vi "Data Format.vi"(9 "Table":refnum<vi>) -> (0 "title":string[](array[string]), 2 "Data":string[](array[string]))   [LabVIEW 2017]
panel:
  out "Error_Description":string
  out "Table":string[][](array[string])
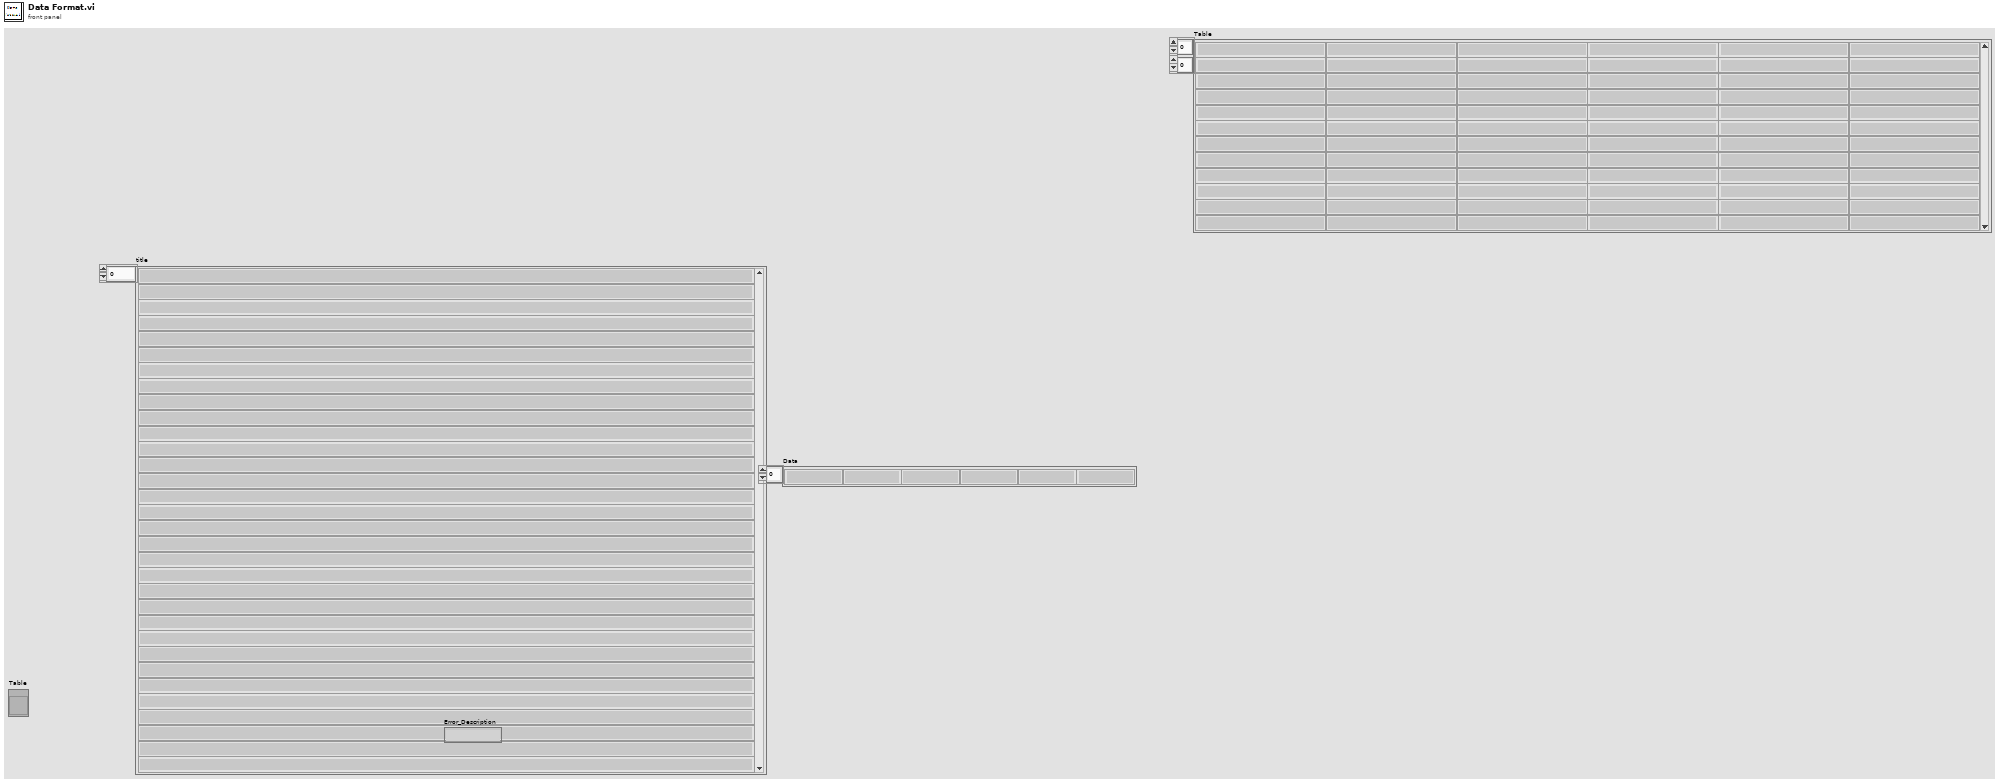
[diagram p1: front panel]
types:
  T1 = typedef "HD Config.ctl" = cluster{" PC":cluster{"PC Address":u8[], "PC Port":i32}, "FCO":cluster{"COM":refnum<visa-resource-name>, "Baudrate":u32}, "DC Power ":cluster{"COM":refnum<visa-resource-name>, "Baudrate":u32}, "PW3336":cluster{"COM":refnum<visa-resource-name>, "Baudrate":u32}, "Lefoo":cluster{"COM":refnum<visa-resource-name>, "Baudrate":u32}, "Tempt&Hum":cluster{"COM":refnum<visa-resource-name>, "Baudrate":u32}, "DIPC":cluster{"COM":refnum<visa-resource-name>}, "Daemon":cluster{"IP Address":string, "Port":u16, "Retry":u16}, "NFC_Cmd":cluster{"COM":refnum<visa-resource-name>, "Baudrate":u32}, "Fail_resume_mode":bool, "GRR":bool, "NFC _Serial":cluster{"COM":refnum<visa-resource-name>, "Baudrate":u32}}
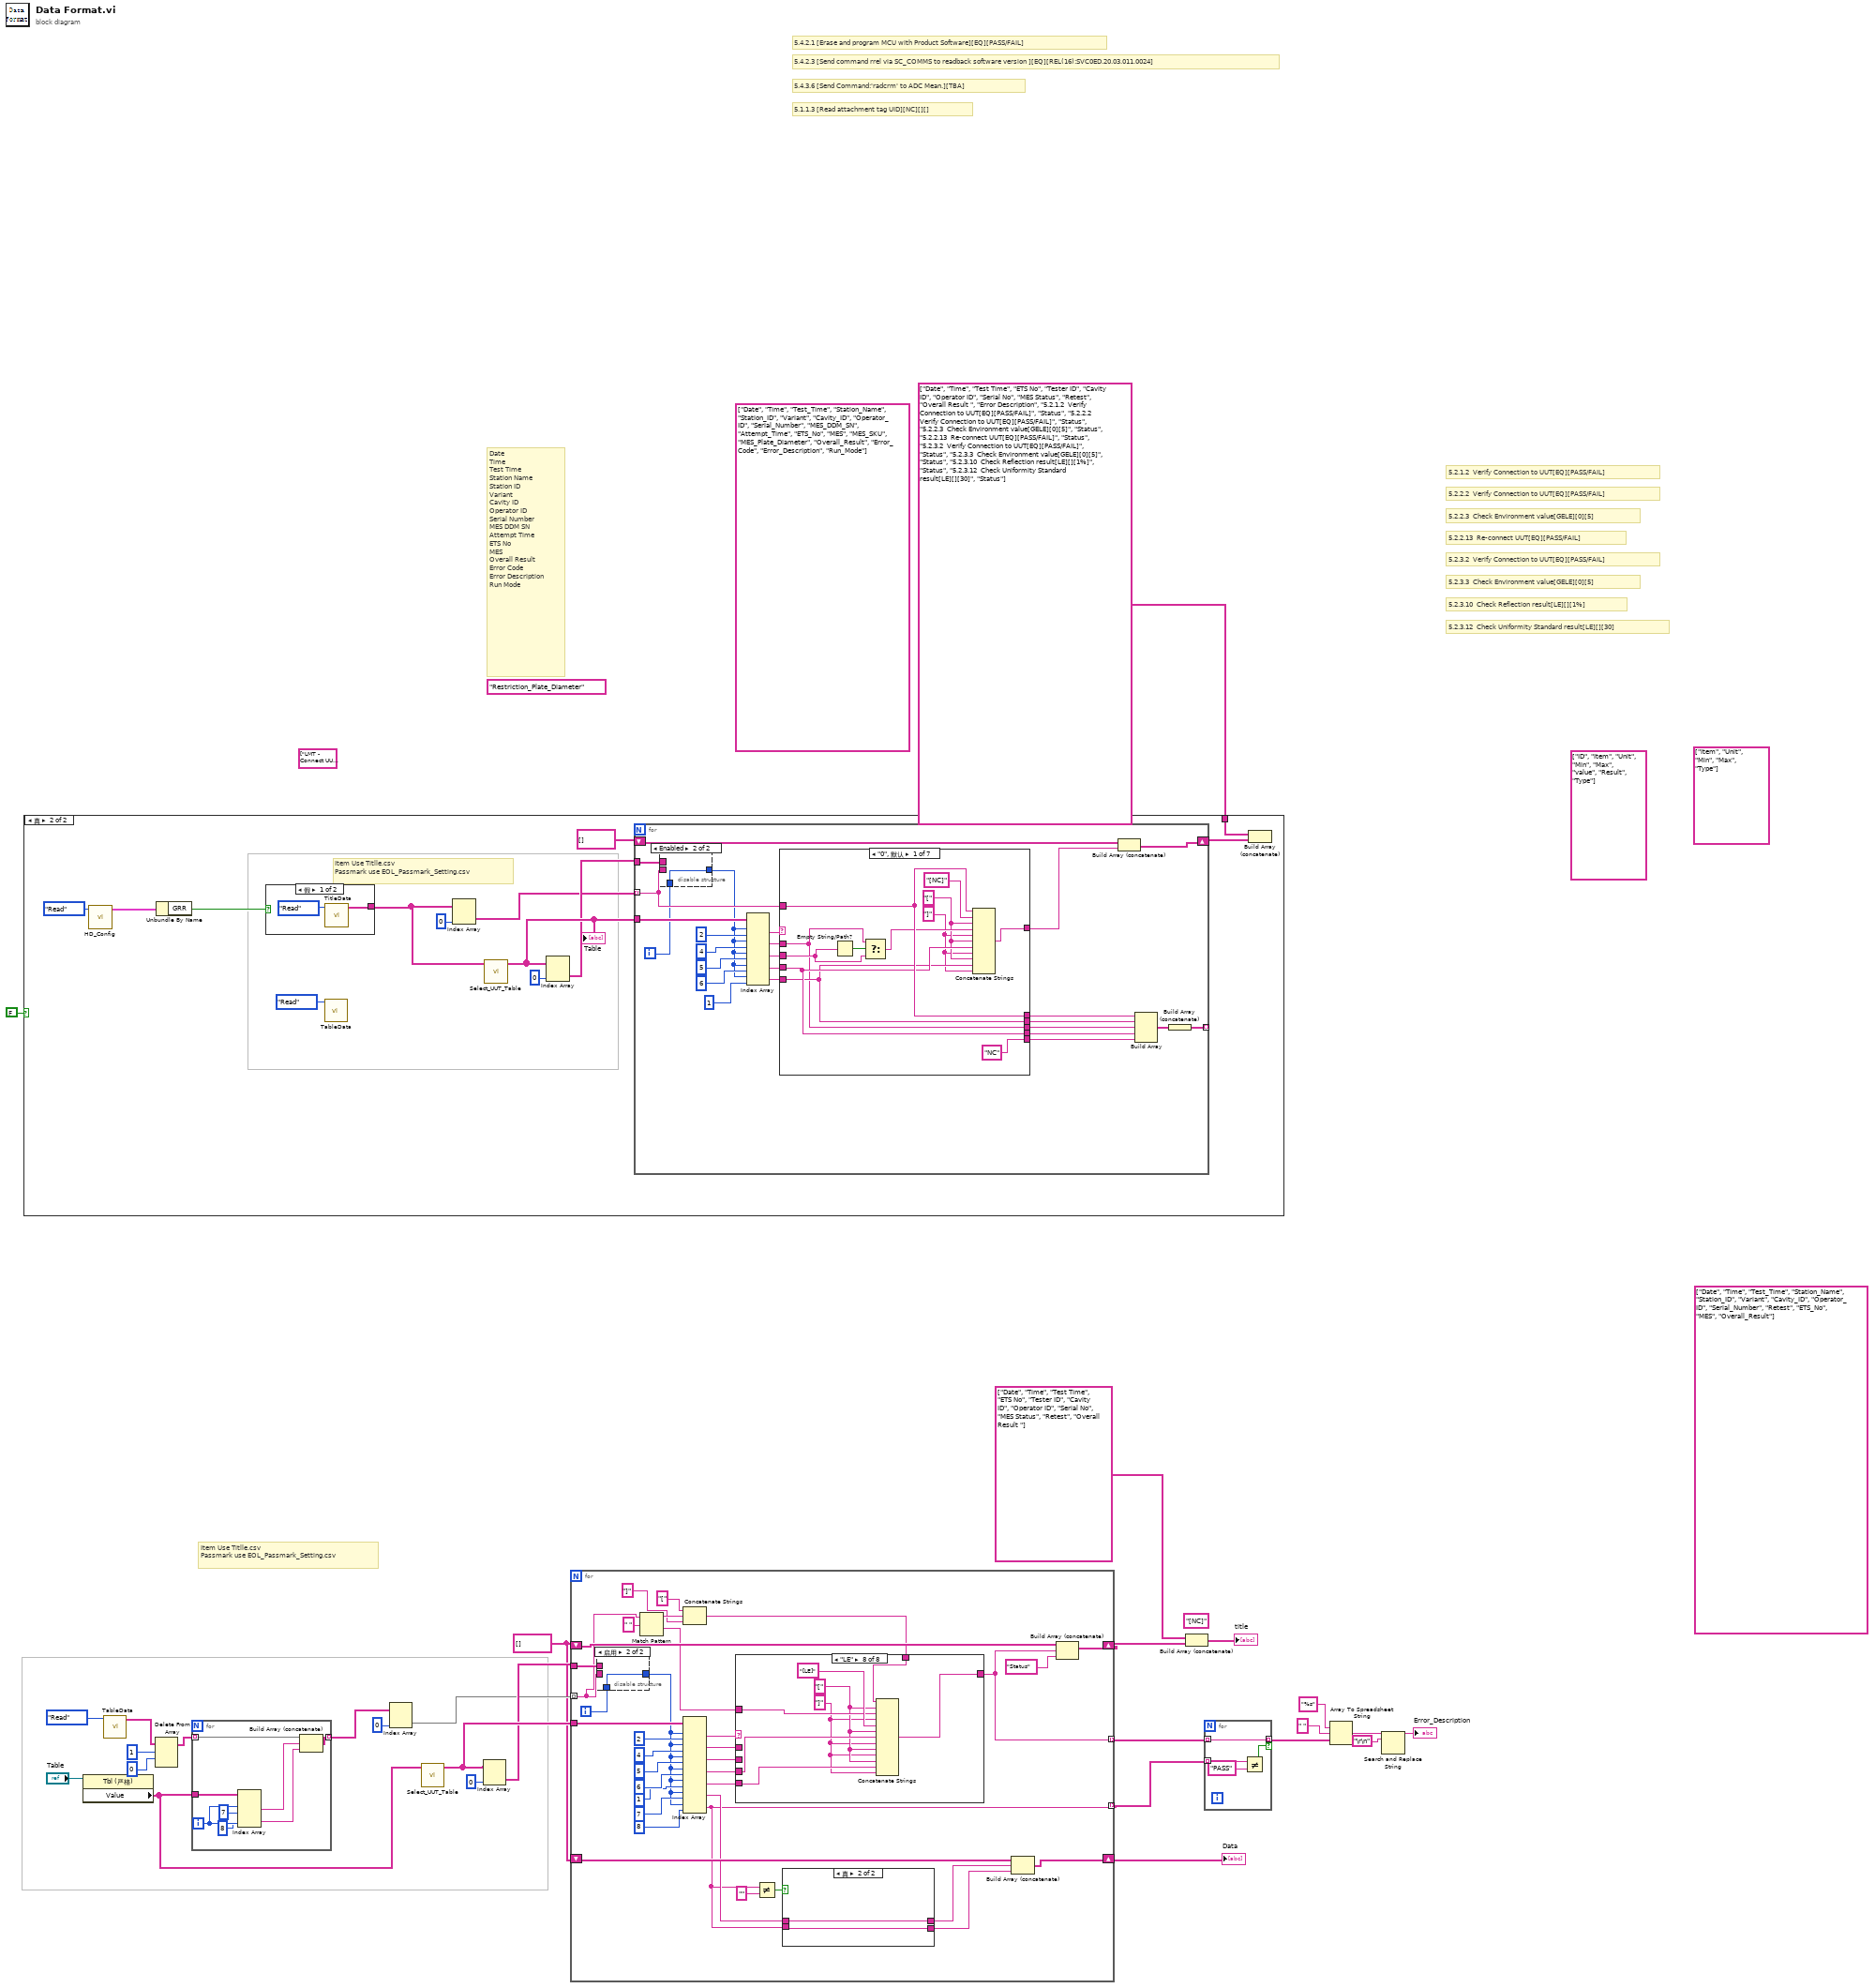
[diagram p0: block diagram]
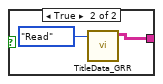
[diagram p3: hidden frame]
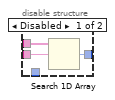
[diagram p4: hidden frame]
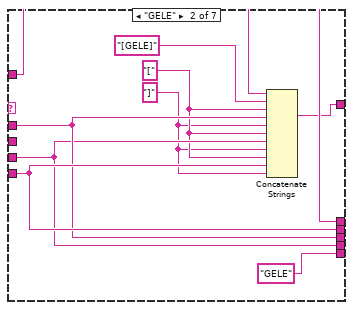
[diagram p5: hidden frame]
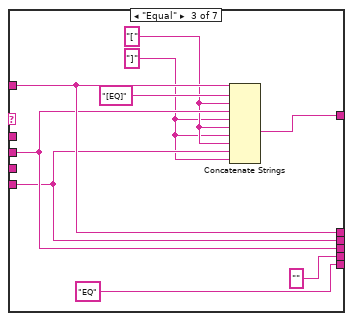
[diagram p6: hidden frame]
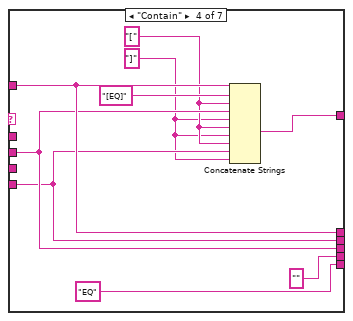
[diagram p7: hidden frame]
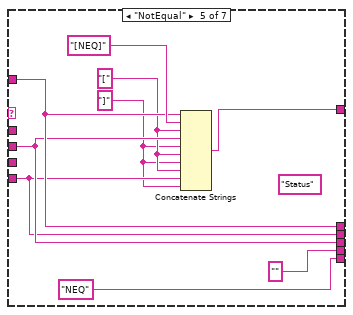
[diagram p8: hidden frame]
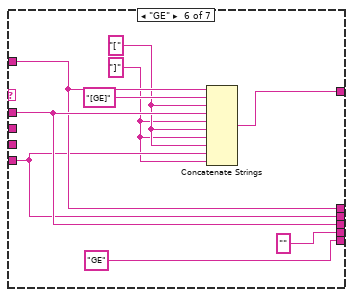
[diagram p9: hidden frame]
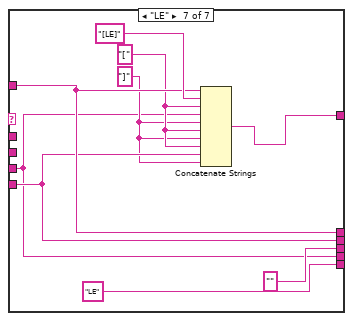
[diagram p10: hidden frame]
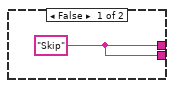
[diagram p11: hidden frame]
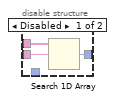
[diagram p12: hidden frame]
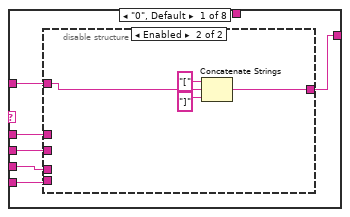
[diagram p13: hidden frame]
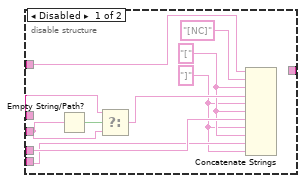
[diagram p14: hidden frame]
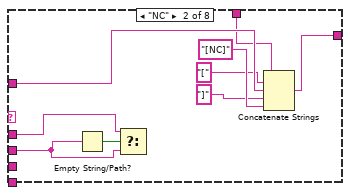
[diagram p15: hidden frame]
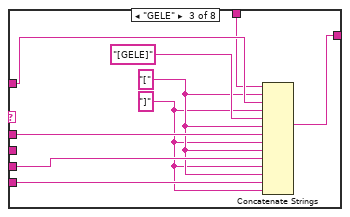
[diagram p16: hidden frame]
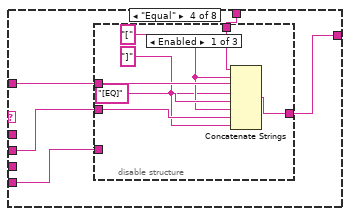
[diagram p17: hidden frame]
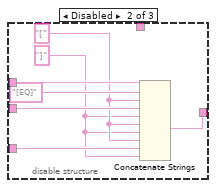
[diagram p18: hidden frame]
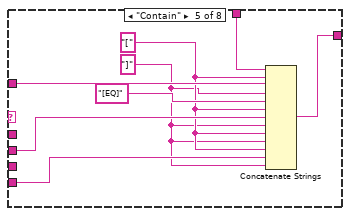
[diagram p20: hidden frame]
diagram:
  (unwired) "[NC]"
  w22 = string[] []
  (unwired) string[] ["Date", "Time", "Test_Time", "Station_Name", "Station_ID", "Variant", "Cavity_ID", "Operator_ID", "Serial_Number", "Retest", "ETS_No", "MES", "Overall_Result"]
  (unwired) "Restriction_Plate_Diameter"
  (unwired) string[] ["ID", "Item", "Unit", "Min", "Max", "value", "Result", "Type"] ("列首字符串[]")
  (unwired) string[] ["LMT - Connect UUT (con COM)", "LMT - Software Version (rrel)", "LMT - Write SKU file (wskuc)", "LMT - SKU file name", "LMT Connect UUT - Error Log", "5.3.2.1 Connect UUT DDM", "Connect UUT DDM - Error Log", "5.3.2.8 Read DDM EOL Timestamp", "5.3.2.8 Read DDM EOL Timestamp - Mode", "5.3.2.8 Read DDM EOL Timestamp - Timestamp", "5.3.2.8 Read DDM EOL Timestamp - Rig ID", "5.3.2.8 Read DDM EOL Timestamp - Passmark ID", "5.3.2.8 Read DDM EOL Timestamp - Passmark Rev", "Read DDM EOL Timestamp - Error Log", "5.3.2.2 Read DDM SW Version before flashing", "5.3.2.2 Software Version before flashing", "Read DDM SW Version before flashing - Error Log", "5.3.2.7 Read Hardware Serial", "Read Hardware Serial - Error Log", "Read DDM SN from UUT", "UUT DDM SN", "Compare Length", "Compare DDM SN with MES SN", "Check DDM SN - Error Log", "5.3.6.2.2 Backup File Data - CAL", "5.3.6.2.2 Backup Data Response - CAL", "5.3.2.3 Flash Firmware Version", "5.3.2.4 Wait Timeout", "5.3.2.5 Check SW Version", "5.3.2.5 Flashing firmware file name", "Flash Firmware Version - Error Log", "5.3.2a.1 Disconnect UUT", "Disconnect UUT - Error Log", "5.3.2a.3 Connect UUT UI", "Connect UUT UI - Error Log", "5.3.2a.4 Flash Firmware Version", "5.3.2a.4 Wait Timeout", "5.3.2a.4 Check SW Version", "5.3.2a.5 Flashing firmware file name", "Flash Firmware Version - Error Log", "5.3.2.6 Read DDM SW Version after flashing", "5.3.2.6 Check DDM SW Version after flashing", "Read DDM SW Version after flashing - Error Log", "5.3.2.10 Set SKU Config Status", "5.3.2.10 Set SKU Config", "5.3.2.10 Set SKU Config File Name", "Set SKU Config - Error Log", "5.3.2.10 Ready Status", "Ready Status - Error Log", "5.3.2.12 Set Device Mode to EOL", "5.3.2.12 DDM EOL mode", "Set Device Mode - Error Log", "5.3.4.34 Wait 1s", "5.3.2.13 DDM Parameter - Voltage", "5.3.2.13 DDM Parameter - Current", "5.3.2.13 DDM Parameter - Power", "5.3.2.13 DDM Parameter - Speed", "5.3.2.13 DDM Parameter - Pressure", "5.3.2.14 Tester Parameter - Voltage", "5.3.2.14 Tester Parameter - Current", "5.3.2.14 Tester Parameter - Power", "5.3.2.14 Tester Parameter - Ambient Pressure", "5.3.2.14 Tester Parameter - Ambient Temperature", "5.3.2.14 Tester Parameter - Pressure Box", "5.3.2.14 Tester Parameter - Reference Ambient Pressure", "5.3.2.15 Calculated Parameter - DDM Pressure Corrected", "5.3.2.15 Calculated Parameter - DDM Real Power", "5.3.2.15 Calculated Parameter - Delta V", "Get and Check Parameter - Error Log", "5.3.3.0 Read BEMF ambient temperature", "5.3.3.0 Calibration Result - eol_cold_bemf_temp", "Read BEMF ambient temperature - Error Log", "5.3.3.0 Set ambient temp to DDM", "5.3.3.0 DDM Ambient Temp", "Set ambient temp to DDM - Error Log", "5.3.4.2 Restriction Plate Diameter", "5.3.4.2 BEMF CAL - Put 13mm Restriction Plate", "Put Restriction Plate - Error Log", "5.3.3.1 Set - Calibrate BEMF both", "5.3.3.1 Get - Calibrate BEMF LSI", "5.3.3.2 Get - Calibration Result - eol_bemf_mp_cold_coef_a", "5.3.3.2 Get - Calibration Result - eol_bemf_mp_cold_coef_b", "5.3.3.2 Get - Calibration Result - eol_bemf_mp_cold_coef_c", "5.3.3.2 Get - Calibration Result - eol_bemf_lsi_cold_ref_coeffs", "5.3.3.2 Get - Calibration Result - eol_bemf_lsi_speed", "5.3.3.2 Get - Calibration Result - eol_bemf_lsi_integral_0", "5.3.3.2 Get - Calibration Result - eol_bemf_lsi_integral_1", "5.3.3.2 Get - Calibration Result - eol_bemf_lsi_integral_2", "5.3.3.2 Get - Calibration Result - eol_cold_bemf", "5.3.3.2 Get - Calibration Result - eol_cold_bemf_fisf", "Get - Calibrate BEMF LSI - Error Log", "5.3.3.3 Finalise Calibration", "5.3.3.4 Wait 1 sec", "Finalise Calibration - Error Log", "5.3.3.1 Get - Calibrate BEMF LSI", "5.3.3.2 Get - Calibration Result - eol_cold_bemf", "5.3.3.2 Get - Calibration Result - eol_cold_bemf_fisf", "5.3.3.2 Compare -Calibration Result - eol_cold_bemf", "5.3.3.2 Compare -Calibration Result - eol_cold_bemf_fisf", "Get & Compare - Calibrate BEMF LSI - Error Log", "5.3.3.3 Reset Power Tune", "5.3.3.4 Reset Power Tune Value", "Reset Power Tune - Error Log", "5.3.3.3 Reset BEMF FISF Calibration", "5.3.3.4 Reset BEMF FISF Calibration Value", "Reset BEMF FISF Calibration - Error Log", "5.3.4.2 ECO - Put 13mm Restriction Plate", "5.3.4.2 Restriction Plate Diameter", "Put Restriction Plate - Error Log", "5.3.4.5 ECO - Motor ON", "5.3.4.5 ECO - Motor ON Mode", "ECO - Motor ON - Error Log", "5.3.4.6 ECO - Motor Speed Stabilisation", "5.3.4.6 ECO - Stabilisation Time", "ECO - Motor Speed Stabilisation - Error Log", "5.3.4.7 ECO - DDM Parameter - Voltage", "5.3.4.7 ECO - DDM Parameter - Current", "5.3.4.7 ECO - DDM Parameter - Power", "5.3.4.7 ECO - DDM Parameter - Measured Power", "5.3.4.7 ECO - DDM Parameter - Speed", "5.3.4.7 ECO - DDM Parameter - Pressure", "5.3.4.7 ECO - DDM Parameter - lsi magnet temp", "5.3.4.7 ECO - DDM Parameter - fisf magnet temp", "5.3.4.7 ECO - DDM Parameter - iir magnet temp", "5.3.4.8 ECO - Tester Parameter - Voltage", "5.3.4.8 ECO - Tester Parameter - Current", "5.3.4.8 ECO - Tester Parameter - Power", "5.3.4.8 ECO - Tester Parameter - Ambient Pressure", "5.3.4.8 ECO - Tester Parameter - Ambient Temperature", "5.3.4.8 ECO - Tester Parameter - Ambient Humidity", "5.3.4.8 ECO - Tester Parameter - Pressure Box", "5.3.4.8 ECO - Tester Parameter - Reference Ambient Pressure", "5.3.4.9 ECO - Calculated Parameter - DDM Pressure Corrected", "5.3.4.9 ECO - Calculated Parameter - DDM Real Power", "5.3.4.9 ECO - Calculated Parameter - Delta V", "5.3.4.9 ECO - Calculated Parameter - Flowrate", "5.3.4.9 ECO - Calculated Parameter - Airwatt", "5.3.4.9 ECO - Formula", "ECO - Get and Check Parameter - Error Log", "PT ECO - Power Tune Mode Status", "PT ECO - Power Tune Set Delta Power Tune", "PT ECO - Power Tune Index", "PT ECO - Power Tune Delta_P", "PT ECO - Power Tune Motor ON Status", "PT ECO - Power Tune Motor ON Mode", "PT ECO - Power Tune Stabilisation Time Status", "PT ECO - Power Tune Stabilisation Delay Time", "PT ECO - DDM Parameter - Voltage", "PT ECO - DDM Parameter - Current", "PT ECO - DDM Parameter - Power", "PT ECO - DDM Parameter - Measured Power", "PT ECO - DDM Parameter - Speed", "PT ECO - DDM Parameter - Pressure", "PT ECO - DDM Parameter - lsi magnet temp", "PT ECO - DDM Parameter - fisf magnet temp", "PT ECO - DDM Parameter - iir magnet temp", "PT ECO - Tester Parameter - Voltage", "PT ECO - Tester Parameter - Current", "PT ECO - Tester Parameter - Power", "PT ECO - Tester Parameter - Ambient Pressure", "PT ECO - Tester Parameter - Ambient Temperature", "PT ECO - Tester Parameter - Ambient Humidity", "PT ECO - Tester Parameter - Pressure Box", "PT ECO - Tester Parameter - Reference Ambient Pressure", "PT ECO - Calculated Parameter - DDM Pressure Corrected", "PT ECO - Calculated Parameter - DDM Real Power", "PT ECO - Calculated Parameter - Delta V", "PT ECO - Calculated Parameter - Flowrate", "PT ECO - Calculated Parameter - Airwatt", "PT ECO - Formula", "PT ECO - Get and Check Parameter - Error Log", "5.3.4.2 BOOST - Put 13mm Restriction Plate", "5.3.4.2 Restriction Plate Diameter", "Put Restriction Plate - Error Log", "5.3.4.5 BOOST - Motor ON", "5.3.4.5 BOOST - Motor ON Mode", "BOOST - Motor ON - Error Log", "5.3.4.6 BOOST - Motor Speed Stabilisation", "5.3.4.6 BOOST - Stabilisation Time", "5.3.4.7 BOOST - DDM Parameter - Voltage", "5.3.4.7 BOOST - DDM Parameter - Current", "5.3.4.7 BOOST - DDM Parameter - Power", "5.3.4.7 BOOST - DDM Parameter - Measured Power", "5.3.4.7 BOOST - DDM Parameter - Speed", "5.3.4.7 BOOST - DDM Parameter - Pressure", "5.3.4.7 BOOST - DDM Parameter - lsi magnet temp", "5.3.4.7 BOOST - DDM Parameter - fisf magnet temp", "5.3.4.7 BOOST - DDM Parameter - iir magnet temp", "5.3.4.8 BOOST - Tester Parameter - Voltage", "5.3.4.8 BOOST - Tester Parameter - Current", "5.3.4.8 BOOST - Tester Parameter - Power", "5.3.4.8 BOOST - Tester Parameter - Ambient Pressure", "5.3.4.8 BOOST - Tester Parameter - Ambient Temperature", "5.3.4.8 BOOST - Tester Parameter - Ambient Humidity", "5.3.4.8 BOOST - Tester Parameter - Pressure Box", "5.3.4.8 BOOST - Tester Parameter - Reference Ambient Pressure", "5.3.4.9 BOOST - Calculated Parameter - DDM Pressure Corrected", "5.3.4.9 BOOST - Calculated Parameter - DDM Real Power", "5.3.4.9 BOOST - Calculated Parameter - Delta V", "5.3.4.9 BOOST - Calculated Parameter - Flowrate", "5.3.4.9 BOOST - Calculated Parameter - Airwatt", "5.3.4.9 BOOST - Formula", "BOOST - Get and Check Parameter - Error Log", "5.3.4.9 BOOST - Check air muscle presence", "5.3.4.9 BOOST - Check air muscle presence Vaule", "BOOST - Check air muscle presence - Error Log", "5.3.4.9 BOOST - Air Muscle Turn Off Status", "5.3.4.9 BOOST - Air Muscle Control", "5.3.3.10 BOOST - Air Muscle Stabilisation Time Status", "5.3.3.10 BOOST - Air Muscle Stabilisation Delay Time", "5.3.4.9 BOOST - Air Muscle Calculated Parameter - Airwatt B", "5.3.4.9 BOOST - Air Muscle Formula", "5.3.4.9 BOOST - Air Muscle Calculate Airwatt Delta", "BOOST - Air Muscle Check - Error Log", "PT BOOST - Power Tune Mode Status", "PT BOOST - Power Tune Set Delta Power Tune", "PT BOOST - Power Tune Index", "PT BOOST - Power Tune Delta_P", "PT BOOST - Power Tune Motor ON Status", "PT BOOST - Power Tune Motor ON Mode", "PT BOOST - Power Tune Stabilisation Time Status", "PT BOOST - Power Tune Stabilisation Delay Time", "PT BOOST - DDM Parameter - Voltage", "PT BOOST - DDM Parameter - Current", "PT BOOST - DDM Parameter - Power", "PT BOOST - DDM Parameter - Measured Power", "PT BOOST - DDM Parameter - Speed", "PT BOOST - DDM Parameter - Pressure", "PT BOOST - DDM Parameter - lsi magnet temp", "PT BOOST - DDM Parameter - fisf magnet temp", "PT BOOST - DDM Parameter - iir magnet temp", "PT BOOST - Tester Parameter - Voltage", "PT BOOST - Tester Parameter - Current", "PT BOOST - Tester Parameter - Power", "PT BOOST - Tester Parameter - Ambient Pressure", "PT BOOST - Tester Parameter - Ambient Temperature", "PT BOOST - Tester Parameter - Ambient Humidity", "PT BOOST - Tester Parameter - Pressure Box", "PT BOOST - Tester Parameter - Reference Ambient Pressure", "PT BOOST - Calculated Parameter - DDM Pressure Corrected", "PT BOOST - Calculated Parameter - DDM Real Power", "PT BOOST - Calculated Parameter - Delta V", "PT BOOST - Calculated Parameter - Flowrate", "PT BOOST - Calculated Parameter - Airwatt", "PT BOOST - Formula", "PT BOOST - Get and Check Parameter - Error Log", "5.3.4.34 Motor OFF", "5.3.4.34 Motor Power", "Motor OFF - Error Log", "5.3.4.34 Wait 1s", "5.3.4.35 Finalise Calibration", "Finalise Calibration - Error Log", "5.3.4.34 ECO - Get AW Calibration Status", "5.3.4.34 ECO - Get AW Calibration value", "5.3.4.34 ECO - Overall Status", "ECO - Get AW Calibration - Error Log", "5.3.4.34 BOOST - Get AW Calibration Status", "5.3.4.34 BOOST - Get AW Calibration value", "5.3.4.34 BOOST - Overall Status", "BOOST - Get AW Calibration - Error Log", "5.3.4.2 MAX - Put 13mm Restriction Plate", "5.3.4.2 Restriction Plate Diameter", "Put Restriction Plate - Error Log", "5.3.4.5 MAX - Motor ON", "5.3.4.5 MAX - Motor ON Mode", "MAX - Motor ON - Error Log", "5.3.4.6 MAX - Motor Speed Stabilisation", "5.3.4.6 MAX - Stabilisation Time", "MAX - Motor Speed Stabilisation - Error Log", "5.3.4.6 Get Average Delta Tmag Status", "5.3.4.6 Get Average Delta Tmag (LSIdelta_FISFdelta_LSItmag_FISFtmag_IIRtmag)", "5.3.4.6 Get Average Delta Tmag LSI", "5.3.4.6 Get Average Delta Tmag FISF", "Get Average Delta Tmag - Error Log", "5.3.4.7 MAX - DDM Parameter - Voltage", "5.3.4.7 MAX - DDM Parameter - Current", "5.3.4.7 MAX - DDM Parameter - Power", "5.3.4.7 MAX - DDM Parameter - Measured Power", "5.3.4.7 MAX - DDM Parameter - Speed", "5.3.4.7 MAX - DDM Parameter - Pressure", "5.3.4.8 MAX - Tester Parameter - Voltage", "5.3.4.8 MAX - Tester Parameter - Current", "5.3.4.8 MAX - Tester Parameter - Power", "5.3.4.8 MAX - Tester Parameter - Ambient Pressure", "5.3.4.8 MAX - Tester Parameter - Ambient Temperature", "5.3.4.8 MAX - Tester Parameter - Ambient Humidity", "5.3.4.8 MAX - Tester Parameter - Pressure Box", "5.3.4.8 MAX - Tester Parameter - Reference Ambient Pressure", "5.3.4.9 MAX - Calculated Parameter - DDM Pressure Corrected", "5.3.4.9 MAX - Calculated Parameter - DDM Real Power", "5.3.4.9 MAX - Calculated Parameter - Delta V", "5.3.4.9 MAX - Calculated Parameter - Flowrate", "5.3.4.9 MAX - Calculated Parameter - Airwatt", "5.3.4.9 MAX - Formula", "MAX - Get and Check Parameter - Error Log", "5.3.3.10 MAX - FISF - Check Average Delta Tmag", "5.3.3.10 MAX - FISF - Check Average Delta Tmag Status", "5.3.3.10 MAX - FISF - BEMF Finetune Result", "BEMF Finetune - Error Log", "MAX tune - Check Airwatts Status", "Calculate Delta Airwatts - MAX tune - Calculate Delta Airwatts", "Calculate Delta Airwatts a - MAX tune - ddm_real_power_a", "Calculate Delta Airwatts b - MAX tune - ddm_real_power_b", "Calculate Delta Airwatts c - MAX tune - Target AW", "Calculate Delta Airwatts d - MAX tune - AW tune extra", "Calculate Delta Airwatts e - MAX tune - Latest AW", "Calculate Delta Airwatts f - MAX tune - correction_factor", "Calculate Delta Airwatts g - MAX tune - P extra", "Calculate Delta Airwatts h - MAX tune - constant power table index", "Calculate Delta Airwatts - MAX tune - Delta P1", "Set AW Tune - MAX tune - Daemon Status", "Set AW Tune - MAX tune - Delta P1 in mW", "Set AW Tune - MAX tune - constant power table index", "Set AW Tune - MAX tune - Drive Mode", "Set AW Tune - MAX tune - Result Airwatt Tune", "5.3.4.5 MAX tune - Motor ON", "5.3.4.5 MAX tune - Motor ON Mode", "5.3.4.6 MAX tune - Motor Speed Stabilisation", "5.3.4.6 MAX tune - Stabilisation Time", "5.3.4.7 MAX tune - DDM Parameter - Voltage", "5.3.4.7 MAX tune - DDM Parameter - Current", "5.3.4.7 MAX tune - DDM Parameter - Power", "5.3.4.7 MAX tune - DDM Parameter - Measured Power", "5.3.4.7 MAX tune - DDM Parameter - Speed", "5.3.4.7 MAX tune - DDM Parameter - Pressure", "5.3.4.7 MAX tune - DDM Parameter - lsi magnet temp", "5.3.4.7 MAX tune - DDM Parameter - fisf magnet temp", "5.3.4.7 MAX tune - DDM Parameter - iir magnet temp", "5.3.4.8 MAX tune - Tester Parameter - Voltage", "5.3.4.8 MAX tune - Tester Parameter - Current", "5.3.4.8 MAX tune - Tester Parameter - Power", "5.3.4.8 MAX tune - Tester Parameter - Ambient Pressure", "5.3.4.8 MAX tune - Tester Parameter - Ambient Temperature", "5.3.4.8 MAX tune - Tester Parameter - Ambient Humidity", "5.3.4.8 MAX tune - Tester Parameter - Pressure Box", "5.3.4.8 MAX tune - Tester Parameter - Reference Ambient Pressure", "5.3.4.9 MAX tune - Calculated Parameter - DDM Pressure Corrected", "5.3.4.9 MAX tune - Calculated Parameter - DDM Real Power", "5.3.4.9 MAX tune - Calculated Parameter - Delta V", "5.3.4.9 MAX tune - Calculated Parameter - Flowrate", "5.3.4.9 MAX tune - Calculated Parameter - Airwatt", "5.3.4.9 MAX tune - Formula", "MAX tune - Get and Check Parameter - Error Log", "MAX finetune - Check Airwatts Status", "Calculate Delta Airwatts - MAX finetune - Calculate Delta Airwatts", "Calculate Delta Airwatts a - MAX finetune - ddm_real_power_a", "Calculate Delta Airwatts b - MAX finetune - ddm_real_power_b", "Calculate Delta Airwatts c - MAX finetune - Target AW", "Calculate Delta Airwatts d - MAX finetune - AW tune extra", "Calculate Delta Airwatts e - MAX finetune - Latest AW", "Calculate Delta Airwatts f - MAX finetune - correction_factor", "Calculate Delta Airwatts g - MAX finetune - P extra", "Calculate Delta Airwatts h - MAX finetune - constant power table index", "Calculate Delta Airwatts - MAX finetune - Delta P2", "Set AW Tune - MAX finetune - Daemon Status", "Set AW Tune - MAX finetune - Delta P2 in mW", "Set AW Tune - MAX finetune - constant power table index", "Set AW Tune - MAX finetune - Drive Mode", "Set AW Tune - MAX finetune - Result Airwatt Finetune", "5.3.4.5 MAX finetune - Motor ON", "5.3.4.5 MAX finetune - Motor ON Mode", "5.3.4.6 MAX finetune - Motor Speed Stabilisation", "5.3.4.6 MAX finetune - Stabilisation Time", "5.3.4.7 MAX finetune - DDM Parameter - Voltage", "5.3.4.7 MAX finetune - DDM Parameter - Current", "5.3.4.7 MAX finetune - DDM Parameter - Power", "5.3.4.7 MAX finetune - DDM Parameter - Measured Power", "5.3.4.7 MAX finetune - DDM Parameter - Speed", "5.3.4.7 MAX finetune - DDM Parameter - Pressure", "5.3.4.7 MAX finetune - DDM Parameter - lsi magnet temp", "5.3.4.7 MAX finetune - DDM Parameter - fisf magnet temp", "5.3.4.7 MAX finetune - DDM Parameter - iir magnet temp", "5.3.4.8 MAX finetune - Tester Parameter - Voltage", "5.3.4.8 MAX finetune - Tester Parameter - Current", "5.3.4.8 MAX finetune - Tester Parameter - Power", "5.3.4.8 MAX finetune - Tester Parameter - Ambient Pressure", "5.3.4.8 MAX finetune - Tester Parameter - Ambient Temperature", "5.3.4.8 MAX finetune - Tester Parameter - Ambient Humidity", "5.3.4.8 MAX finetune - Tester Parameter - Pressure Box", "5.3.4.8 MAX finetune - Tester Parameter - Reference Ambient Pressure", "5.3.4.9 MAX finetune - Calculated Parameter - DDM Pressure Corrected", "5.3.4.9 MAX finetune - Calculated Parameter - DDM Real Power", "5.3.4.9 MAX finetune - Calculated Parameter - Delta V", "5.3.4.9 MAX finetune - Calculated Parameter - Flowrate", "5.3.4.9 MAX finetune - Calculated Parameter - Airwatt", "5.3.4.9 MAX finetune - Formula", "MAX finetune - Get and Check Parameter - Error Log", "5.3.3.10 Check Derate Status", "5.3.3.10 Check Derate Result", "Check Derate Status - Get and Check Parameter - Error Log", "5.3.4.6 Get Delta Tmag After Tuned Status", "5.3.4.6 Delta Tmag FISF", "5.3.4.6 FISF Tmag", "5.3.4.6 IIR Tmag", "Get Delta Tmag After Tuned - Error Log", "5.3.3.10 Get Hot BEMF Status", "5.3.3.10 Get Hot BEMF Result", "Get Hot BEMF Status - Get and Check Parameter - Error Log", "5.3.4.34 Motor OFF", "5.3.4.34 Motor Power", "Motor OFF - Error Log", "5.3.4.34 Wait 1s", "Wait - Error Log", "5.3.3.10 Get DDM Pressure Status", "5.3.3.10 DDM Pressure", "5.3.3.10 Tester Ambient Pressure", "5.3.3.10 Calculate delta Pressure", "Get DDM Pressure Status - Get and Check Parameter - Error Log", "5.3.4.35 Finalise Calibration", "5.3.4.36 Wait 1 sec", "Finalise Calibration - Error Log", "5.3.3.0 Get Cold BEMF Status", "5.3.3.0 Get Cold BEMF - eol_cold_bemf_fisf", "5.3.3.0 Calculate & Check Delta BEMF", "Get Cold BEMF fisf - Error Log", "5.3.4.34 Get AW Calibration Status", "5.3.4.34 Delta P Airwatts Value", "5.3.4.34 Get Airwatts Tune Index 2", "5.3.4.34 Compare Result", "Get AW Calibration - Error Log", "5.3.3.0 Read DDM ambient temperature", "5.3.3.0 Calibration Result - eol_cold_bemf_temp", "Read BEMF ambient temperature - Error Log", "5.3.3.0 Set ambient temp to DDM", "5.3.3.0 DDM Ambient Temp", "Set ambient temp to DDM - Error Log", "5.3.5.1 Reset Task Detect - LL", "5.3.5.1 Reset Task Detect - HL", "5.3.5.1 Reset Task Detect - LH", "5.3.5.1 Reset Task Detect - HH", "5.3.5.1 Reset eol inlet blockage", "5.3.5.2 LL - Put 30mm Restriction Plate", "5.3.5.2 Restriction Plate Diameter", "Put Restriction Plate - Error Log", "5.3.5.4 LL - A2 mode Motor ON", "5.3.5.4 LL - A2 mode Motor Power", "LL -A2 mode Motor ON - Error Log", "5.3.5.5 LL - Motor Speed Stabilisation", "5.3.5.5 LL - Stabilisation Time", "LL - Motor Speed Stabilisation - Error Log", "5.3.5.6 LL - DDM Parameter - Voltage", "5.3.5.6 LL - DDM Parameter - Current", "5.3.5.6 LL - DDM Parameter - Power", "5.3.5.6 LL - DDM Parameter - Measured Power", "5.3.5.6 LL - DDM Parameter - Speed", "5.3.5.6 LL - DDM Parameter - Pressure", "5.3.5.7 LL - Tester Parameter - Voltage", "5.3.5.7 LL - Tester Parameter - Current", "5.3.5.7 LL - Tester Parameter - Power", "5.3.5.7 LL - DDM Real Power", "5.3.5.7 LL - Get and Check Parameter - Error Log", "5.3.5.8 LL - Calibrate Task Detect LL", "5.3.5.8 LL - Set Calibrate Task Detect LL", "5.3.5.8 LL - Calibrate Task Detect - Error Log", "5.3.5.4 HL - BOOST mode Motor ON", "5.3.5.4 HL - BOOST mode Motor Power", "HL - BOOST mode Motor ON - Error Log", "5.3.5.5 HL - Motor Speed Stabilisation", "5.3.5.5 HL - Stabilisation Time", "HL - Motor Speed Stabilisation - Error Log", "5.3.5.6 HL - DDM Parameter - Voltage", "5.3.5.6 HL - DDM Parameter - Current", "5.3.5.6 HL - DDM Parameter - Power", "5.3.5.6 HL - DDM Parameter - Measured Power", "5.3.5.6 HL - DDM Parameter - Speed", "5.3.5.6 HL - DDM Parameter - Pressure", "5.3.5.7 HL - Tester Parameter - Voltage", "5.3.5.7 HL - Tester Parameter - Current", "5.3.5.7 HL - Tester Parameter - Power", "5.3.5.7 HL - DDM Real Power", "5.3.5.7 HL - Get and Check Parameter - Error Log", "5.3.5.8 HL - Calibrate Task Detect HL", "5.3.5.8 HL - Set Calibrate Task Detect HL", "5.3.5.8 HL - Calibrate Task Detect - Error Log", "5.3.5.15 Motor OFF", "5.3.5.15 Motor Power", "Motor OFF - Error Log", "5.3.5.15 Wait 1s", "Wait - Error Log", "5.3.5.2 LH - Put 16mm Restriction Plate", "5.3.5.2 Restriction Plate Diameter", "Put Restriction Plate - Error Log", "5.3.5.4 LH -A2 mode Motor ON", "5.3.5.4 LH - A2 mode Motor Power", "LH - A2 mode Motor ON - Error Log", "5.3.5.5 LH - Motor Speed Stabilisation", "5.3.5.5 LH - Stabilisation Time", "LH - Motor Speed Stabilisation - Error Log", "5.3.5.6 LH - DDM Parameter - Voltage", "5.3.5.6 LH - DDM Parameter - Current", "5.3.5.6 LH - DDM Parameter - Power", "5.3.5.6 LH - DDM Parameter - Measured Power", "5.3.5.6 LH - DDM Parameter - Speed", "5.3.5.6 LH - DDM Parameter - Pressure", "5.3.5.7 LH - Tester Parameter - Voltage", "5.3.5.7 LH - Tester Parameter - Current", "5.3.5.7 LH - Tester Parameter - Power", "5.3.5.7 LH - DDM Real Power", "5.3.5.7 LH - Get and Check Parameter - Error Log", "5.3.5.8 LH - Calibrate Task Detect LH", "5.3.5.8 LH - Set Calibrate Task Detect LH", "5.3.5.8 LH - Calibrate Task Detect - Error Log", "5.3.5.4 HH - BOOST mode Motor ON", "5.3.5.4 HH - BOOST mode Motor Power", "HH - BOOST mode Motor ON - Error Log", "5.3.5.5 HH - Motor Speed Stabilisation", "5.3.5.5 HH - Stabilisation Time", "HH - Motor Speed Stabilisation - Error Log", "5.3.5.6 HH - DDM Parameter - Voltage", "5.3.5.6 HH - DDM Parameter - Current", "5.3.5.6 HH - DDM Parameter - Power", "5.3.5.6 HH - DDM Parameter - Measured Power", "5.3.5.6 HH - DDM Parameter - Speed", "5.3.5.6 HH - DDM Parameter - Pressure", "5.3.5.7 HH - Tester Parameter - Voltage", "5.3.5.7 HH - Tester Parameter - Current", "5.3.5.7 HH - Tester Parameter - Power", "5.3.5.7 HH - DDM Real Power", "5.3.5.7 HH - Get and Check Parameter - Error Log", "5.3.5.8 HH - Calibrate Task Detect HH", "5.3.5.8 HH - Set Calibrate Task Detect HH", "5.3.5.8 HH - Calibrate Task Detect - Error Log", "5.3.5.29 Wait 1s", "Wait - Error Log", "Inlet Blockage Calibration - Motor ON", "Inlet Blockage Calibration - Motor Power", "Inlet Blockage Calibration - Motor ON - Error Log", "Inlet Blockage Calibration - Motor Speed Stabilisation", "Inlet Blockage Calibration - Stabilisation Time", "Inlet Blockage Calibration - Motor Speed Stabilisation - Error Log", "Inlet Blockage Calibration - DDM Parameter - Voltage", "Inlet Blockage Calibration - DDM Parameter - Current", "Inlet Blockage Calibration - DDM Parameter - Power", "Inlet Blockage Calibration - DDM Parameter - Measured Power", "Inlet Blockage Calibration - DDM Parameter - Speed", "Inlet Blockage Calibration - DDM Parameter - Pressure", "Inlet Blockage Calibration - DDM Parameter - lsi magnet temp", "Inlet Blockage Calibration - DDM Parameter - fisf magnet temp", "Inlet Blockage Calibration - DDM Parameter - iir magnet temp", "Inlet Blockage Calibration - Tester Parameter - Voltage", "Inlet Blockage Calibration - Tester Parameter - Current", "Inlet Blockage Calibration - Tester Parameter - Power", "Inlet Blockage Calibration - DDM Real Power", "Inlet Blockage Calibration - Get and Check Parameter - Error Log", "5.3.5.30 Set Calibrate Inlet Blockage", "5.3.5.30 Calibrate Inlet Blockage Value", "5.3.5.31 Calibrate Inlet Blockage - Wait 1s", "Calibrate Inlet Blockage - Error Log", "5.3.5.15 Motor OFF", "5.3.5.15 Motor Power", "Motor OFF - Error Log", "5.3.5.32 Wait 1s", "Wait - Error Log", "5.3.5.35 Get Calibration Inlet Blockage", "5.3.5.35 Calibration Inlet Blockage", "Get Calibration Inlet Blockage - Error Log", "5.3.3.0 Set ambient temp to DDM", "5.3.3.0 DDM Ambient Temp", "Set ambient temp to DDM - Error Log", "5.3.5.33 Finalise Calibration", "5.3.5.34 Wait 1 sec", "Finalise Calibration - Error Log", "5.3.5.35 Get Task Detect LL", "5.3.5.35 Get Task Detect HL", "5.3.5.35 Get Task Detect LH", "5.3.5.35 Get Task Detect HH", "Get Task Detect - Error Log", "5.3.5.35 Get Calibration Inlet Blockage", "5.3.5.35 Calibration Inlet Blockage", "5.3.5.35 Calibration eol cold bemf temp", "5.3.5.35 Compare Task Detect LL", "5.3.5.35 Compare Task Detect HL", "5.3.5.35 Compare Task Detect LH", "5.3.5.35 Compare Task Detect HH", "5.3.5.35 Compare Calibration Inlet Blockage", "5.3.5.35 Compare Calibration eol cold bemf temp", "Compare Task Detect Inlet Blockage - Error Log", "5.3.6.1.2 GOOD UNIT - Clear EEPROM Error Log", "GOOD UNIT - Clear EEPROM Error Log - Error Log", "5.3.6.1.3 GOOD UNIT - Write Product Timestamp", "5.3.6.1.3 GOOD UNIT - Write Product Timestamp - Mode", "5.3.6.1.3 GOOD UNIT - Write Product Timestamp - Timestamp", "5.3.6.1.3 GOOD UNIT - Write Product Timestamp - Rig ID", "5.3.6.1.3 GOOD UNIT - Write Product Timestamp - Passmark ID", "5.3.6.1.3 GOOD UNIT - Write Product Timestamp - Passmark Rev", "GOOD UNIT - Write Product Timestamp - Error Log", "5.3.2.12 GOOD UNIT - Set Device Mode to PROD", "5.3.2.12 GOOD UNIT - DDM PROD mode", "GOOD UNIT - Set Device Mode - Error Log", "5.3.6.1.6 GOOD UNIT - Wait 1s Delay", "GOOD UNIT - Delay - Error Log", "5.3.2.8 GOOD UNIT - Read DDM PROD Timestamp", "5.3.2.8 GOOD UNIT - Read DDM PROD Timestamp - Mode", "5.3.2.8 GOOD UNIT - Read DDM PROD Timestamp - Timestamp", "5.3.2.8 GOOD UNIT - Read DDM PROD Timestamp - Rig ID", "5.3.2.8 GOOD UNIT - Read DDM PROD Timestamp - Passmark ID", "5.3.2.8 GOOD UNIT - Read DDM PROD Timestamp - Passmark Rev", "5.3.2.8 Compare - Read DDM PROD Timestamp", "5.3.2.8 Compare - Read DDM PROD Timestamp - Mode", "5.3.2.8 Compare - Read DDM PROD Timestamp - Timestamp", "5.3.2.8 Compare - Read DDM PROD Timestamp - Rig ID", "5.3.2.8 Compare - Read DDM PROD Timestamp - Passmark ID", "5.3.2.8 Compare - Read DDM PROD Timestamp - Passmark Rev", "GOOD UNIT - Read DDM PROD Timestamp - Error Log", "5.3.6.1.7 GOOD UNIT - Backup File Data", "5.3.6.1.7 GOOD UNIT - Backup File Data  - Error Log", "5.3.2.7 GOOD UNIT - Check Security Bit", "GOOD UNIT - Check Security Bit - Error Log", "5.3.6.1.8 GOOD UNIT - Set Calibration Lock", "GOOD UNIT - Set Calibration Lock - Error Log", "5.3.6.1.9 GOOD UNIT - Disconnect UUT", "GOOD UNIT - Disconnect UUT - Error Log", "5.3.6.2.2 NG UNIT - Read NVM Error", "NG UNIT - Read NVM Error - Error Log", "5.3.2.12 NG UNIT - DDM FCT mode", "5.3.2.12 NG UNIT - DDM FCT mode", "NG UNIT - Set Device Mode - Error Log", "5.3.6.2.2 NG UNIT - Backup File Data - CAL", "5.3.6.2.2 NG UNIT - Backup File Data - ERROR", "5.3.6.2.2 NG UNIT - Backup File Data - USAGE", "NG UNIT - Backup File Data - Error Log", "5.3.6.2.4 NG UNIT - Disconnect UUT", "NG UNIT - Disconnect UUT - Error Log"] ("数组 2")
  (unwired) string[] ["Item", "Unit", "Min", "Max", "Type"] ("列首字符串[]")
  (unwired) string[] ["Date", "Time", "Test_Time", "Station_Name", "Station_ID", "Variant", "Cavity_ID", "Operator_ID", "Serial_Number", "MES_DDM_SN", "Attempt_Time", "ETS_No", "MES", "MES_SKU", "MES_Plate_Diameter", "Overall_Result", "Error_Code", "Error_Description", "Run_Mode"]
  # "Item Use Titlle.csv\nPassmark use EOL_Passmark_Setting.csv"
  # "5.2.3.12  Check Uniformity Standard result[LE][][30]"
  # "5.2.3.10  Check Reflection result[LE][][1%]"
  # "5.2.3.3  Check Environment value[GELE][0][5]"
  # "5.2.3.2  Verify Connection to UUT[EQ][PASS/FAIL]"
  # "5.2.2.13  Re-connect UUT[EQ][PASS/FAIL]"
  # "5.2.2.3  Check Environment value[GELE][0][5]"
  # "5.2.2.2  Verify Connection to UUT[EQ][PASS/FAIL]"
  # "5.2.1.2  Verify Connection to UUT[EQ][PASS/FAIL]"
  # "5.4.3.6 [Send Command:'radcrm' to ADC Mean.][TBA]"
  # "5.4.2.3 [Send command rrel via SC_COMMS to readback software version ][EQ][REL(16):SVC0ED.20.03.011.0024]"
  # "5.4.2.1 [Erase and program MCU with Product Software][EQ][PASS/FAIL]"
  # "5.1.1.3 [Read attachment tag UID][NC][][]"
  # "Date\nTime\nTest Time\nStation Name\nStation ID\nVariant\nCavity ID\nOperator ID\nSerial Number\nMES DDM SN\nAttempt Time\nETS No\nMES\nOverall Result\nError Code\nError Description\nRun Mode"
  n1 = case shown="真" FALSE {
    tunnel: string[] ["Date", "Time", "Test Time", "ETS No", "Tester ID", "Cavity ID", "Operator ID", "Serial No", "MES Status", "Retest", "Overall Result ", "Error Description", "5.2.1.2  Verify Connection to UUT[EQ][PASS/FAIL]", "Status", "5.2.2.2  Verify Connection to UUT[EQ][PASS/FAIL]", "Status", "5.2.2.3  Check Environment value[GELE][0][5]", "Status", "5.2.2.13  Re-connect UUT[EQ][PASS/FAIL]", "Status", "5.2.3.2  Verify Connection to UUT[EQ][PASS/FAIL]", "Status", "5.2.3.3  Check Environment value[GELE][0][5]", "Status", "5.2.3.10  Check Reflection result[LE][][1%]", "Status", "5.2.3.12  Check Uniformity Standard result[LE][][30]", "Status"] ("title") -> [_ w29]
    frame False {
    }
    frame True {
      # "Item Use Titlle.csv\nPassmark use EOL_Passmark_Setting.csv"
      n2 = call "HD_Config.vi"("Step"=enum16{"Initial", "Write", "Read"}."Read") -> ("HD Config out"=w31:T1)  [unwired: 9 in, 1 out]
      n3 = Unbundle By Name(w31) -> ("GRR"=w30:bool)
      n4 = case shown="假" w30 {
        tunnel: [w42 w44] -> w34
        frame False {
          n5 = call "TitleData.vi"("Step"=enum16{"Initial", "Write", "Read"}."Read") -> ("Tabledata Out"=w42:string[][])  [unwired: 9 in, 1 out]
        }
        frame True {
          n6 = call "TitleData_GRR.vi"("Step"=enum16{"Initial", "Write", "Read"}."Read") -> ("Tabledata Out"=w44:string[][])  [unwired: 9 in, 1 out]
        }
      }
      n7 = call "TableData.vi"("Step"=enum16{"Initial", "Write", "Read"}."Read") -> ()  [unwired: 9 in, 2 out]
      n8 = Index Array "Index Array"(array=w34, index (col)=0 ("禁用的索引 (列)")) -> (element=w35:string[])  [unwired: 1 in]
      n9 = call "Select_UUT_Table.vi"("all Table"=w34) -> ("Table"=w41:string[][])  [unwired: 9 in, 1 out]
      "Table" <- w41
      n10 = Index Array(array=w41, index (col)=0 ("禁用的索引 (列)")) -> (element=w39:string[])  [unwired: 1 in]
      n11 = for {
        tunnel: w35 -> [w58] mode=indexing
        tunnel: w41 -> [w69]
        tunnel: w39 -> [w70]
        shift-right: [w59] -> w37
        shift-left: string[] [] -> [w60]
        tunnel: [w51] -> _ mode=indexing
        i -> [w46]
        n12 = disable-structure shown="Enabled" {
          disable-tunnel: w70 -> [w73 _]
          disable-tunnel: w58 -> [w72 _]
          disable-tunnel: [w71 w74] -> w48
          disable-tunnel: w46 -> [_ w74]
          frame Disabled {
            n13 = Search 1D Array(1D array=w73, element=w72) -> (index of element=w71:i32)  [unwired: 1 in]
          }
          frame Enabled {
          }
        }
        n14 = Index Array(array=w69, index (row) #1=w48, index (col) #1=2 ("禁用的索引 (列)"), index (row) #2=w48, index (col) #2=4 ("禁用的索引 (列)"), index (row) #3=w48, index (col) #3=5 ("禁用的索引 (列)"), index (row) #4=w48, index (col) #4=6 ("禁用的索引 (列)"), index (row) #5=w48, index (col) #5=1 ("索引 (列)")) -> (element #1=w67:string, element #2=w63:string, element #3=w62:string, element #4=w61:string, element #5=w49:string)
        n15 = case shown="\"0\", 默认" w67 {
          tunnel: w63 -> [w78 w90 _ _ _ w130 _]
          tunnel: w62 -> [w79 _ w101 w110 w119 _ _]
          tunnel: w61 -> [w82 w89 _ _ _ _ w132]
          tunnel: [w83 w92 w99 w108 w117 w126 w136] -> w47
          tunnel: w58 -> [w85 w94 w103 w112 w121 w129 w139]
          tunnel: [w85 w94 w103 w112 w121 w129 w139] -> w57
          tunnel: [w78 w90 w101 w110 w119 w130 "" ("String")] -> w56
          tunnel: [w82 w89 "" ("String") "" ("String") "" ("String") "" ("String") w132] -> w55
          tunnel: ["NC" "GELE" "EQ" "EQ" "NEQ" "GE" "LE"] -> w54
          tunnel: [w81 w91 w98 w107 w115 w125 w135] -> w52
          tunnel: w49 -> [w81 w91 w98 w107 w115 w125 w135]
          frame "0", Default {
            w75 = "]" ("字符串")
            w76 = "[" ("字符串")
            n16 = Empty String/Path?(string/path=w79) -> (empty?=w80:bool)
            n17 = Select(t=w78, s=w80, f=w79) -> (s? t:f=w77:string)
            n18 = Concatenate Strings(w85, "[NC]", w76, w77, w75, w76, w82, w75, w76, w81, w75) -> (w83:string)
          }
          frame "GELE" {
            w87 = "]" ("字符串")
            w88 = "[" ("字符串")
            n19 = Concatenate Strings(w94, "[GELE]", w88, w90, w87, w88, w89, w87, w88, w91, w87) -> (w92:string)
          }
          frame "Equal" {
            w96 = "]" ("字符串")
            w97 = "[" ("字符串")
            n20 = Concatenate Strings(w103, "[EQ]", w97, w101, w96, w97, w96, w97, w98, w96) -> (w99:string)
          }
          frame "Contain" {
            w105 = "]" ("字符串")
            w106 = "[" ("字符串")
            n21 = Concatenate Strings(w112, "[EQ]", w106, w110, w105, w106, w105, w106, w107, w105) -> (w108:string)
          }
          frame "NotEqual" {
            (unwired) "Status" ("元素")
            w114 = "]" ("字符串")
            w116 = "[" ("字符串")
            n22 = Concatenate Strings(w121, "[NEQ]", w116, w119, w114, w116, w114, w116, w115, w114) -> (w117:string)
          }
          frame "GE" {
            w123 = "]" ("字符串")
            w124 = "[" ("字符串")
            n23 = Concatenate Strings(w129, "[GE]", w124, w130, w123, w124, w123, w124, w125, w123) -> (w126:string)
          }
          frame "LE" {
            w133 = "]" ("字符串")
            w134 = "[" ("字符串")
            n24 = Concatenate Strings(w139, "[LE]", w134, w132, w133, w134, w133, w134, w135, w133) -> (w136:string)
          }
        }
        n25 = Build Array (concatenate)(w60, w47) -> (w59:string[])
        n26 = Build Array ("创建数组")(w57, w52, w56, w55, w54) -> (w53:string[])
        n27 = Build Array (concatenate) ("创建数组")(w53) -> (w51:string[])
      }
      n28 = Build Array (concatenate)(w29, w37) -> ()  [unwired: 1 out]
    }
  }
  n29 = property class="Tbl (严格)"(reference="Table") -> ("Value"=w1:string[][])  [unwired: 1 in, 2 out]
  n30 = call "TableData.vi"("Step"=enum16{"Initial", "Write", "Read"}."Read") -> ("Tabledata Out"=w5:string[][])  [unwired: 9 in, 1 out]
  n31 = Delete From Array(array=w5, length=1, index (row)=0) -> (array with subset deleted=w2:string[][])  [unwired: 1 in, 1 out]
  n32 = for {
    tunnel: w2 -> [w147] mode=indexing
    tunnel: w1 -> [w148]
    tunnel: [w146] -> w6 mode=indexing
    i -> [w145]
    n33 = Index Array(array=w148, index (row) #1=w145, index (col) #1=7 ("index"), index (row) #2=w145, index (col) #2=8 ("index")) -> (element #1=w142:string, element #2=w141:string)
    n34 = Build Array (concatenate)(w147, w142, w141) -> (w146:string[])
  }
  n35 = Index Array "Index Array"(array=w6, index (col)=0 ("禁用的索引 (列)")) -> (element=w23:string[])  [unwired: 1 in]
  n36 = call "Select_UUT_Table.vi"("all Table"=w1) -> ("Table"=w28:string[][])  [unwired: 9 in, 1 out]
  n37 = Index Array(array=w28, index (col)=0 ("禁用的索引 (列)")) -> (element=w26:string[])  [unwired: 1 in]
  n38 = for {
    tunnel: w23 -> [w158] mode=indexing
    tunnel: w28 -> [w182]
    tunnel: w26 -> [w183]
    shift-right: [w172] -> w25
    shift-left: w22 -> [w173]
    shift-right: [w165] -> w21
    shift-left: w22 -> [w166]
    tunnel: [w162] -> w20 mode=indexing
    tunnel: [w151] -> w19 mode=indexing
    i -> [w169]
    n39 = disable-structure shown="启用" {
      disable-tunnel: w183 -> [w189 _]
      disable-tunnel: w158 -> [w188 _]
      disable-tunnel: [w187 w190] -> w164
      disable-tunnel: w169 -> [_ w190]
      frame Disabled {
        n40 = Search 1D Array(1D array=w189, element=w188) -> (index of element=w187:i32)  [unwired: 1 in]
      }
      frame Enabled {
      }
    }
    n41 = Match Pattern(string=w158, regular expression=" ") -> (before substring=w161:string, after substring=w157:string)  [unwired: 1 in, 2 out]
    n42 = Concatenate Strings("[" ("字符串"), w161, "]" ("字符串")) -> (w156:string)
    n43 = Index Array(array=w182, index (row) #1=w164, index (col) #1=2 ("禁用的索引 (列)"), index (row) #2=w164, index (col) #2=4 ("禁用的索引 (列)"), index (row) #3=w164, index (col) #3=5 ("禁用的索引 (列)"), index (row) #4=w164, index (col) #4=6 ("禁用的索引 (列)"), index (row) #5=w164, index (col) #5=1 ("索引 (列)"), index (row) #6=w164, index (col) #6=7 ("disabled index (col)"), index (row) #7=w164, index (col) #7=8 ("disabled index (col)")) -> (element #1=w180:string, element #2=w176:string, element #3=w175:string, element #4=w174:string, element #5=w170:string, element #6=w152:string, element #7=w151:string)
    n44 = case shown="\"LE\"" w180 {
      tunnel: w176 -> [w193 w214 w224 _ _ _ w270 _]
      tunnel: w175 -> [w194 w215 _ w232 w253 w261 _ _]
      tunnel: w174 -> [w196 _ w223 _ _ _ _ w275]
      tunnel: [w191 w217 w226 w231 w252 w260 w268 w277] -> w162
      tunnel: w157 -> [w192 w218 w227 w233 w254 w262 w269 w278]
      tunnel: w170 -> [w195 _ w225 w230 w251 w259 w267 w276]
      tunnel: w156 -> [_ w211 w220 w229 w248 w256 w264 w272]
      frame "0", Default {
        n45 = disable-structure shown="Enabled" {
          disable-tunnel: w196 -> [w205 _]
          disable-tunnel: w195 -> [w204 _]
          disable-tunnel: w194 -> [w202 _]
          disable-tunnel: w193 -> [w201 _]
          disable-tunnel: w192 -> [w197 w210]
          disable-tunnel: [_ w209] -> w191
          frame Disabled {
            w198 = "]" ("字符串")
            w199 = "[" ("字符串")
            n46 = Empty String/Path?(string/path=w202) -> (empty?=w203:bool)
            n47 = Select(t=w201, s=w203, f=w202) -> (s? t:f=w200:string)
            n48 = Concatenate Strings(w197, "[NC]", w199, w200, w198, w199, w205, w198, w199, w204, w198) -> ()  [unwired: 1 out]
          }
          frame Enabled {
            n49 = Concatenate Strings("[" ("string"), w210, "]" ("string")) -> (w209:string)
          }
        }
      }
      frame "NC" {
        n50 = Empty String/Path?(string/path=w215) -> (empty?=w216:bool)
        n51 = Select(t=w214, s=w216, f=w215) -> ()  [unwired: 1 out]
        n52 = Concatenate Strings(w211, "[" ("字符串"), w218, "]" ("字符串"), "[NC]") -> (w217:string)
      }
      frame "GELE" {
        w221 = "]" ("字符串")
        w222 = "[" ("字符串")
        n53 = Concatenate Strings(w220, w222, w227, w221, "[GELE]", w222, w224, w221, w222, w223, w221, w222, w225, w221) -> (w226:string)
      }
      frame "Equal" {
        n54 = disable-structure shown="Enabled" {
          disable-tunnel: w233 -> [w239 w246 _]
          disable-tunnel: w232 -> [w238 w245 _]
          disable-tunnel: [w237 w244 _] -> w231
          disable-tunnel: w230 -> [_ w243 _]
          disable-tunnel: w229 -> [w234 _ _]
          frame Enabled {
            w235 = "]" ("字符串")
            w236 = "[" ("字符串")
            n55 = Concatenate Strings(w234, w236, w239, w235, "[EQ]", w236, w238, w235) -> (w237:string)
          }
          frame Disabled {
            w241 = "]" ("字符串")
            w242 = "[" ("字符串")
            n56 = Concatenate Strings(w246, "[EQ]", w242, w245, w241, w242, w241, w242, w243, w241) -> (w244:string)
          }
          frame Disabled {
          }
        }
      }
      frame "Contain" {
        w249 = "]" ("字符串")
        w250 = "[" ("字符串")
        n57 = Concatenate Strings(w248, w250, w254, w249, "[EQ]", w250, w253, w249, w250, w249, w250, w251, w249) -> (w252:string)
      }
      frame "NotEqual" {
        w257 = "]" ("字符串")
        w258 = "[" ("字符串")
        n58 = Concatenate Strings(w256, w258, w262, w257, "[NEQ]", w258, w261, w257, w258, w257, w258, w259, w257) -> (w260:string)
      }
      frame "GE" {
        w265 = "]" ("字符串")
        w266 = "[" ("字符串")
        n59 = Concatenate Strings(w264, w266, w269, w265, "[GE]", w266, w270, w265, w266, w265, w266, w267, w265) -> (w268:string)
      }
      frame "LE" {
        w273 = "]" ("字符串")
        w274 = "[" ("字符串")
        n60 = Concatenate Strings(w272, w274, w278, w273, "[LE]", w274, w275, w273, w274, w273, w274, w276, w273) -> (w277:string)
      }
    }
    n61 = Not Equal?(x=w151, y="") -> (x != y?=w153:bool)
    n62 = case shown="真" w153 {
      tunnel: w152 -> [_ w186]
      tunnel: [w184 w186] -> w150
      tunnel: [w184 w185] -> w149
      tunnel: w151 -> [_ w185]
      frame False {
        w184 = "Skip" ("y")
      }
      frame True {
      }
    }
    n63 = Build Array (concatenate)(w166, w150, w149) -> (w165:string[])
    n64 = Build Array (concatenate)(w173, w162, "Status" ("element")) -> (w172:string[])
  }
  "Data" <- w21
  n65 = Build Array (concatenate)(string[] ["Date", "Time", "Test Time", "ETS No", "Tester ID", "Cavity ID", "Operator ID", "Serial No", "MES Status", "Retest", "Overall Result "] ("title_beforedata"), w25) -> (→"title":string[])
  n66 = for {
    tunnel: [w283] -> w14 mode=indexing if=w280
    tunnel: w20 -> [w283] mode=indexing
    tunnel: w19 -> [w282] mode=indexing
    n67 = Not Equal?(x=w282, y="PASS") -> (x != y?=w280:bool)
  }
  n68 = Array To Spreadsheet String(delimiter (Tab)=" ", array=w14, 3:"%s" ("delimiter (Tab)")) -> (spreadsheet string=w16:string)
  n69 = Search and Replace String(input string=w16, search string="\r\n") -> (result string=→"Error_Description":string)  [unwired: 6 in, 3 out]
